vi "PolarMeterCheck.vi"(1 "错误输入（无错误）":errorcluster) -> (2 "通信正常？":bool, 4 "错误输出":errorcluster)   [LabVIEW 2018]
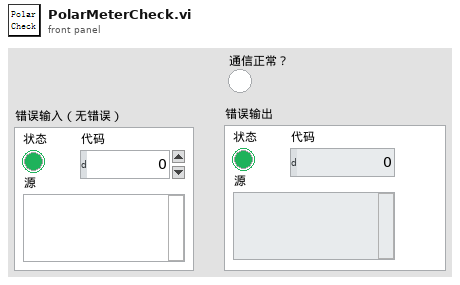
[diagram p1: front panel]
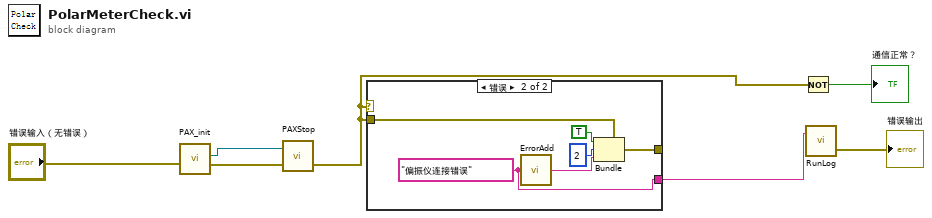
[diagram p0: block diagram]
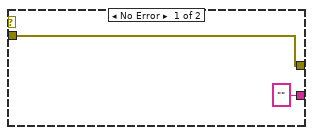
[diagram p2: hidden frame]
diagram:
  n1 = call "PAX_init.vi"("Error In"="错误输入（无错误）") -> ("error out"=w4:errorcluster, "偏振测量仪VISA"=w5:refnum<visa-resource-name>)  [unwired: 9 in]
  n2 = call "PAXStop.vi"("error in"=w4, "VISA 输入"=w5) -> ("error out"=w1:errorcluster)  [unwired: 1 in]
  n3 = case shown="错误" w1 {
    tunnel: w1 -> [w9 w12]
    tunnel: [w9 w11] -> _
    tunnel: ["" w10] -> w6
    frame No Error {
    }
    frame Error {
      w10 = "偏振仪连接错误" ("source")
      n4 = call "ErrorAdd.vi"("source"=w10) -> ("Errorout Souce"=w13:string)
      n5 = Bundle(cluster=w12, "status"=TRUE, "code"=2, "source"=w13) -> (w11:errorcluster)
    }
  }
  n6 = Not(x=w1) -> (.not. x?=→"通信正常？":bool)
  n7 = call "RunLog.vi"("Message"=w6) -> ("error out"=→"错误输出":errorcluster)  [unwired: 2 in]
